vi "Run.vi"(8 "error in (no error)":errorcluster caption="entrée d'erreur (pas d'erreur)", 9 "Y":string[][](array[string]), 10 "X":string[][](array[string]), 11 "Paired_euclidean_distances.lvclass":refnum<class "Paired_euclidean_distances.lvclass">) -> (0 "error out":errorcluster caption="sortie d'erreur", 2 "Data":T1, 3 "Paired_euclidean_distances.lvclass":refnum<class "Paired_euclidean_distances.lvclass">)   [LabVIEW 2020, in "Paired_euclidean_distances.lvclass"]
doc: "Returns :\n\n- distances : ndarray (n_samples, )"
uses:
  Paired_euclidean_distances.lvclass
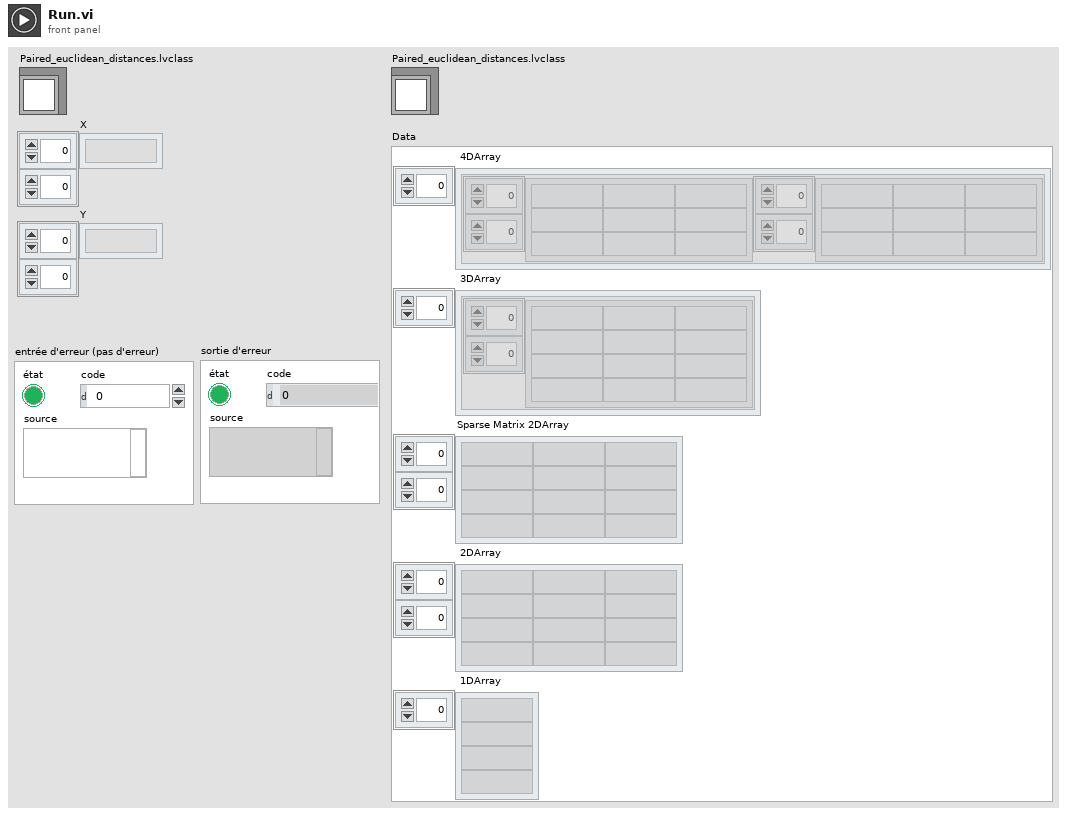
[diagram p1: front panel]
types:
  T1 = cluster{" 4DArray":cluster{"1":string[][], "2":string[][]}[], " 3DArray":cluster{"Tableau":string[][]}[], "Sparse Matrix 2DArray":string[][], " 2DArray":string[][], " 1DArray":string[]}
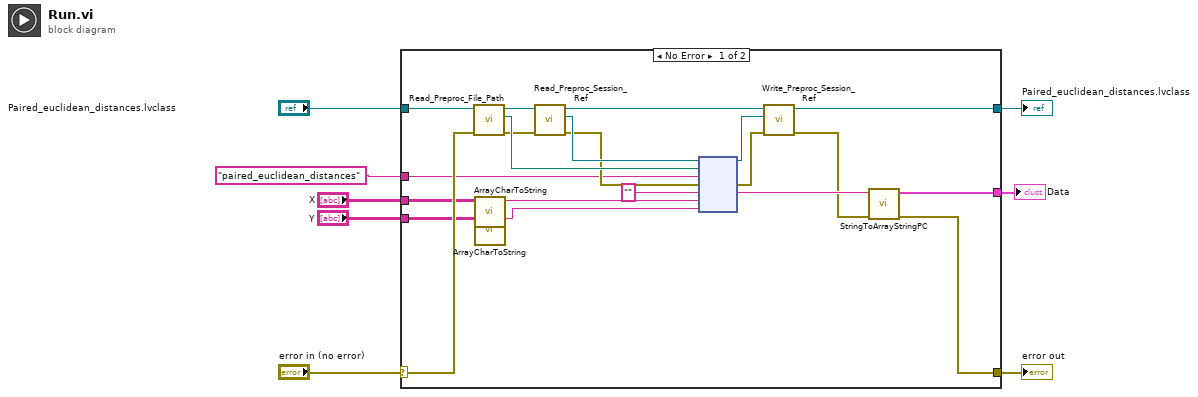
[diagram p0: block diagram]
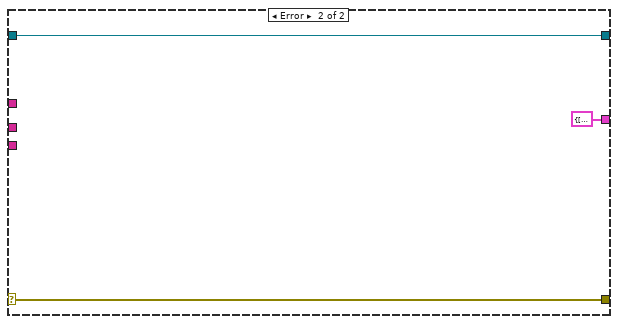
[diagram p2: hidden frame]
diagram:
  n1 = case shown="No Error" "error in (no error)" {
    selector: "error in (no error)" -> [w20 w32]
    tunnel: [w11 w32] -> w7
    tunnel: [w9 w31] -> w5
    tunnel: "Paired_euclidean_distances.lvclass" -> [w18 w31]
    tunnel: "paired_euclidean_distances" ("Fonction") -> [w19 _]
    tunnel: "X" -> [w17 _]
    tunnel: "Y" -> [w16 _]
    tunnel: [w10 T1 {" 4DArray"=[], " 3DArray"=[], "Sparse Matrix 2DArray"=[], " 2DArray"=[], " 1DArray"=[]} ("Data")] -> w1
    frame No Error {
      n2 = call-dynamic "Read_Preproc_File_Path.vi"("error in (no error)"=w20, "Python in"=w18) -> ("error out"=w24:errorcluster, "File_Path"=w27:path, "Python out"=w29:refnum<class "Paired_euclidean_distances.lvclass">)  [unwired: 7 in]
      n3 = call "ArrayCharToString.vi"("TAB"=w17) -> ("Instruction"=w15:string)  [unwired: 10 in]
      n4 = call "ArrayCharToString.vi"("TAB"=w16) -> ("Instruction"=w14:string)  [unwired: 10 in]
      n5 = call-dynamic "Read_Preproc_Session_Ref.vi"("error in (no error)"=w24, "Python in"=w29) -> ("error out"=w25:errorcluster, "Session_ref"=w26:refnum<k35>, "Python out"=w28:refnum<class "Paired_euclidean_distances.lvclass">)  [unwired: 7 in]
      n6 = node(w26, w27, w19, w25, "", w15, w14) -> (w21:refnum<k35>, w23:errorcluster, w13:string)  [unwired: 2 in, 2 out]
      n7 = call-dynamic "Write_Preproc_Session_Ref.vi"("error in (no error)"=w23, "Session_ref"=w21, "Python in"=w28) -> ("error out"=w12:errorcluster, "Python out"=w9:refnum<class "Paired_euclidean_distances.lvclass">)  [unwired: 7 in]
      n8 = call "StringToArrayStringPC.vi"("sortie d'erreur"=w12, "Return value"=w13) -> ("sortie d'erreur"=w11:errorcluster, "Data"=w10:T1)  [unwired: 8 in]
    }
    frame Error {
    }
  }
  "error out" <- w7
  "Paired_euclidean_distances.lvclass" <- w5
  "Data" <- w1
